vi "Get Ingredients.vi"(8 "error in (no error)":errorcluster, 11 "Metal in":refnum<class "Metal.lvclass">) -> (0 "error out":errorcluster, 2 "Ingredients":T1[](array[typedef]), 3 "Metal out":refnum<class "Metal.lvclass">)   [LabVIEW 2020, in "Metal.lvclass"]
uses:
  Metal.lvclass
  Item/Ingredient.ctl
  Item/Item.lvclass
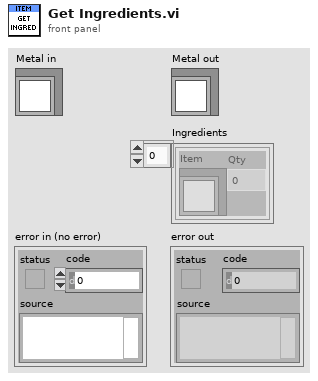
[diagram p1: front panel]
types:
  T1 = typedef "Item.lvclass/Ingredient.ctl" = cluster{"Item":refnum<class "Item.lvclass">, "Qty":dbl}
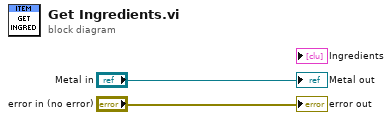
[diagram p0: block diagram]
diagram:
  "error out" <- "error in (no error)"
  "Metal out" <- "Metal in"
